vi "SQLite Backup Old Calibration Value.vi"(6 "backup/Delete":enum16{"Backup", "Delete"}(ring), 7 "Main":string="0", 8 "error in (no error)":errorcluster, 11 "VariableName":string) -> (0 "error out":errorcluster)   [LabVIEW 2017, in "SQLite.lvclass"]
doc: "保存校准的结果值,.\n2015-11-03 16:29:50\nBy：蒋松\nEmail：jiangsong@outlook.com\nSina: @sushu1051"
uses:
  SQLite.lvclass
  SQLiteFileName.ctl
  TabelFullName.ctl
  <vilib>/Utility/error.llb/Trim Whitespace.vi
  <userlib>/_OpenG.lib/array/array.llb/Remove Duplicates from 1D Array (String)__ogtk.vi
  <userlib>/LabSQL/LabSQL.lvlib
panel:
  out "Result Set":string[][](table) caption="Result Set (from first statement with results)"
  # "insert 之前要先删除所有的就的校准值。\n2015-11-03 16:45:40\nBy：蒋松\nEmail：jiangsong@outlook.com\nSina: @sushu1051"
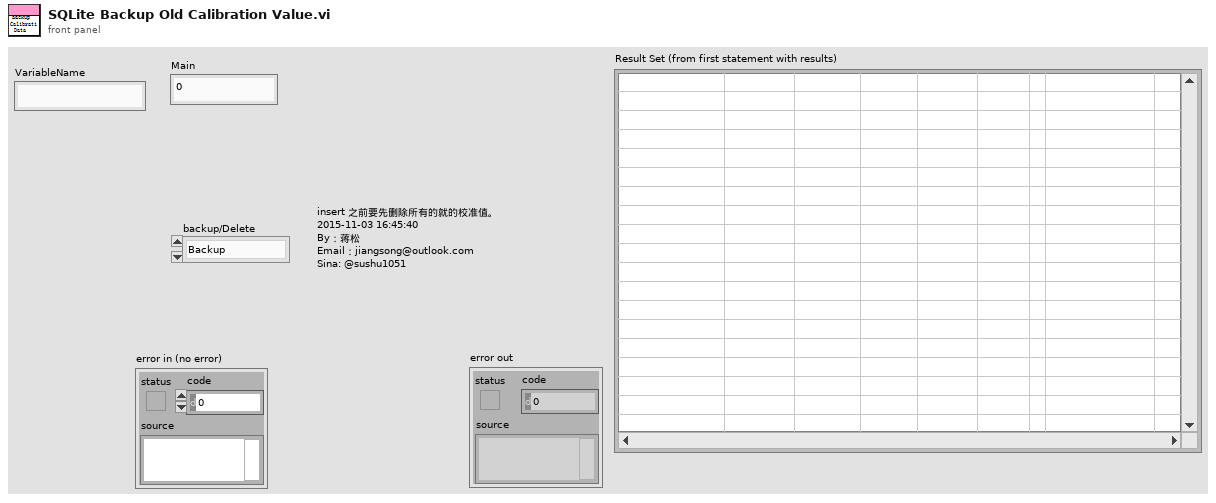
[diagram p1: front panel]
types:
  T1 = typedef "SQLite.lvclass/TabelFullName.ctl" = string
  T2 = typedef "SQLite.lvclass/SQLiteFileName.ctl" = string
  T3 = enum32{"invalid app kind", "Development System", "Run Time System", "Student Edition", "Embedded LabVIEW", "Evaluation", "Custom"}
  T4 = enum32{"Invalid", "Standard", "Closed", "Hidden", "Minimized", "Maximized"}
  T5 = enum16{"Other", "SQL2008", "SQLite", "Access", "MySQL"}
  T6 = cluster{"Core":cluster{"Current VI Reference":refnum<vi>, "Close Panel on Exit?":bool}}
  T7 = cluster{"Current VI Reference":refnum<vi>, "Close Panel on Exit?":bool}
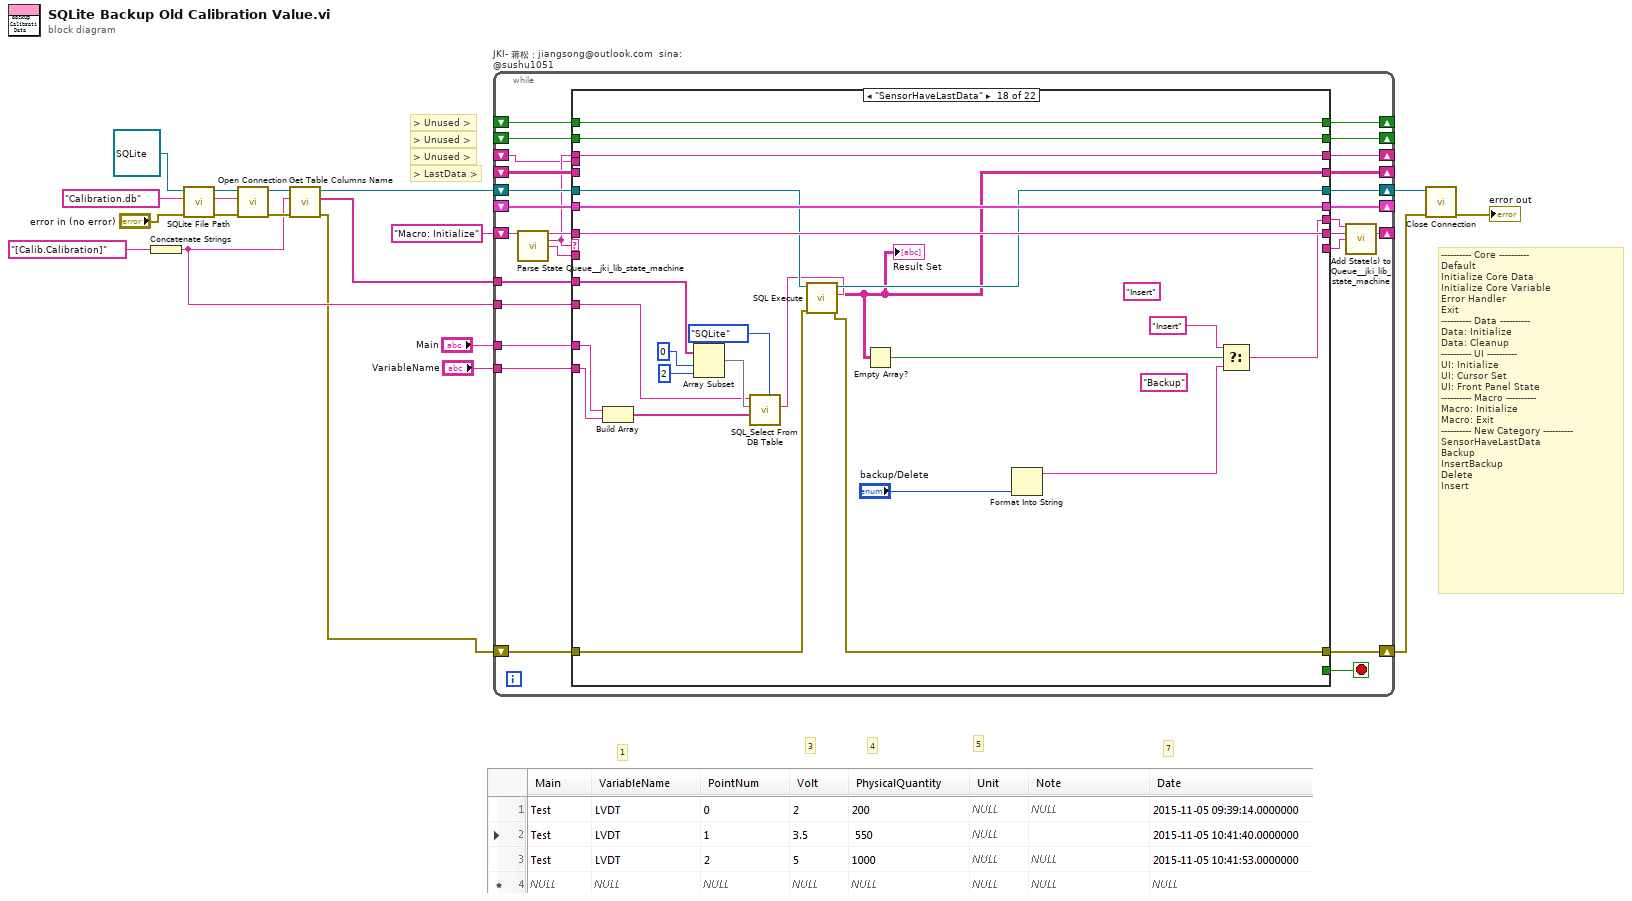
[diagram p0: block diagram]
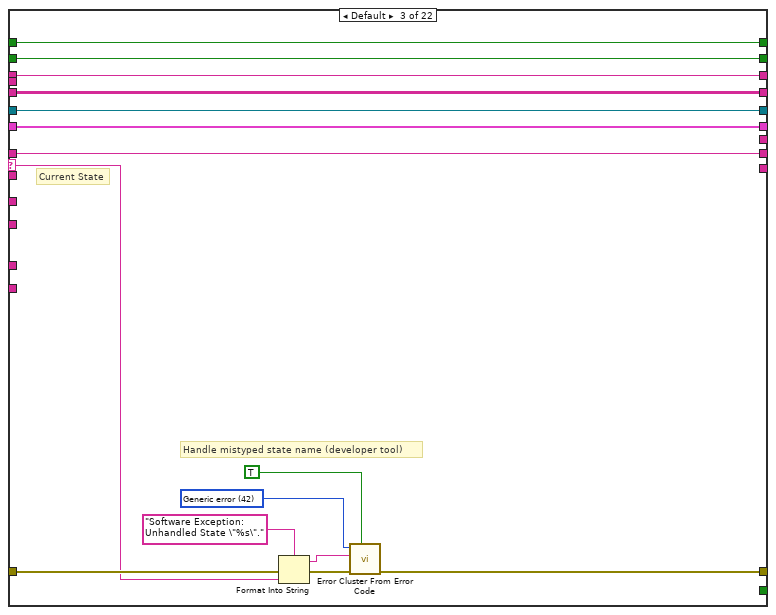
[diagram p4: hidden frame]
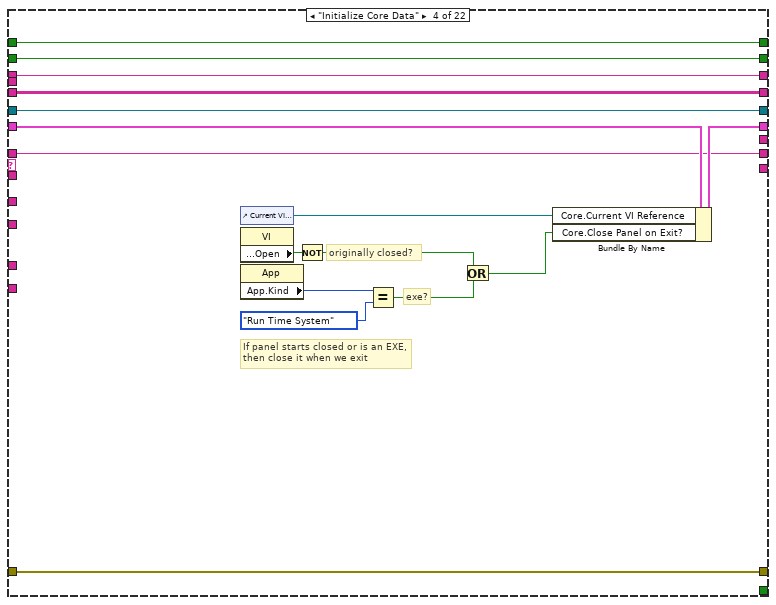
[diagram p5: hidden frame]
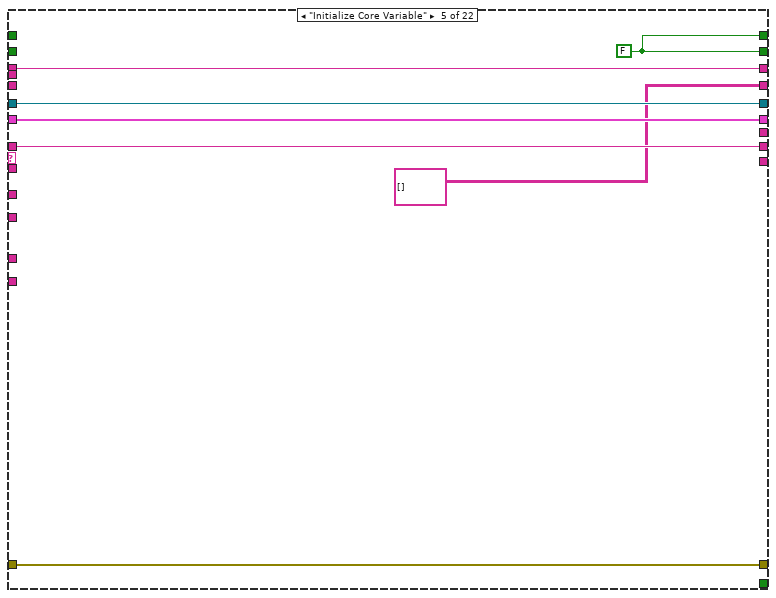
[diagram p6: hidden frame]
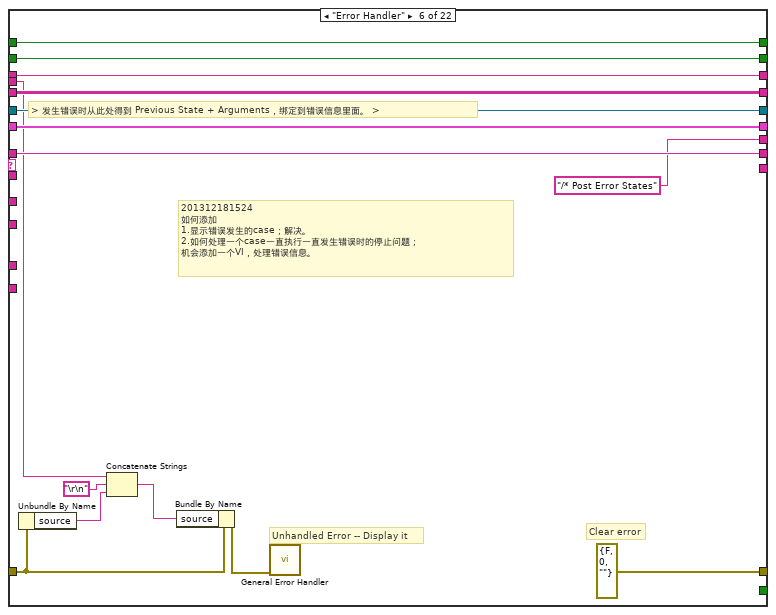
[diagram p7: hidden frame]
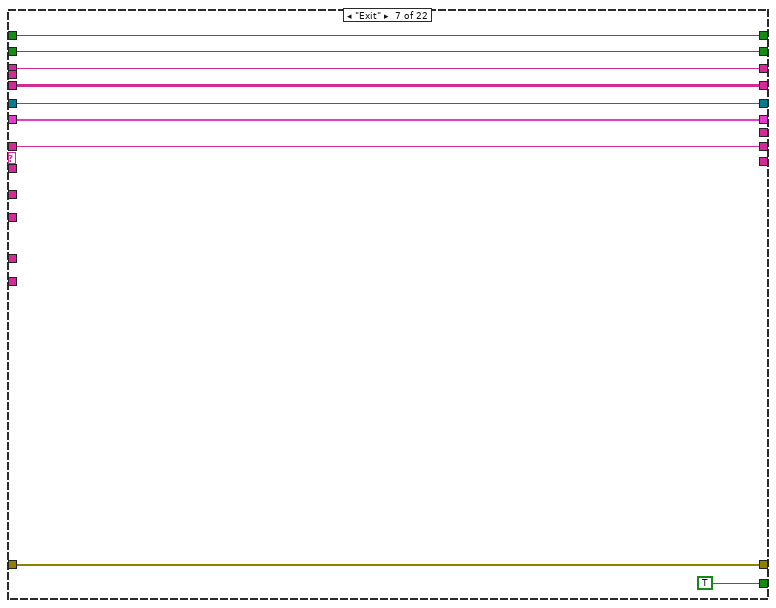
[diagram p8: hidden frame]
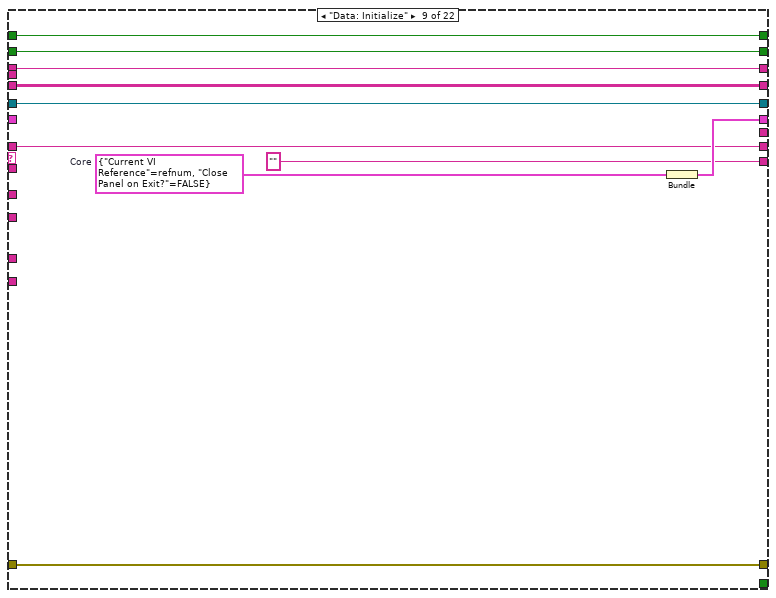
[diagram p10: hidden frame]
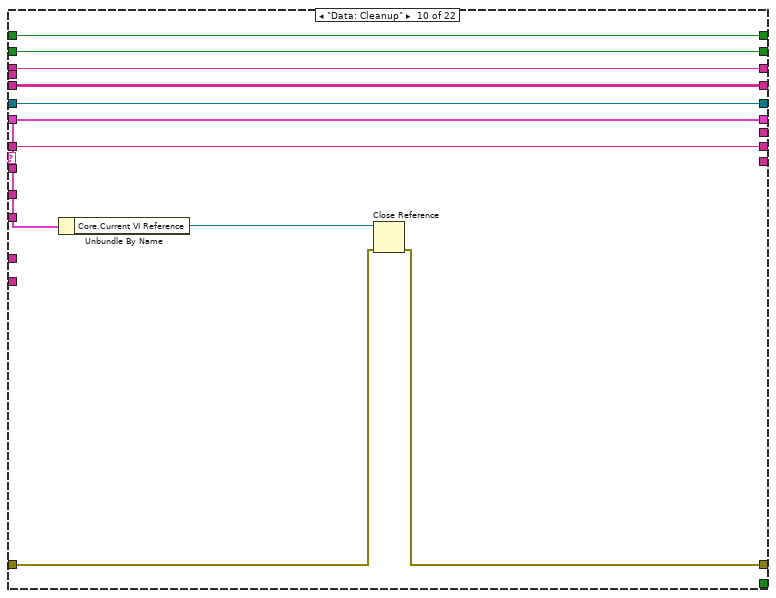
[diagram p11: hidden frame]
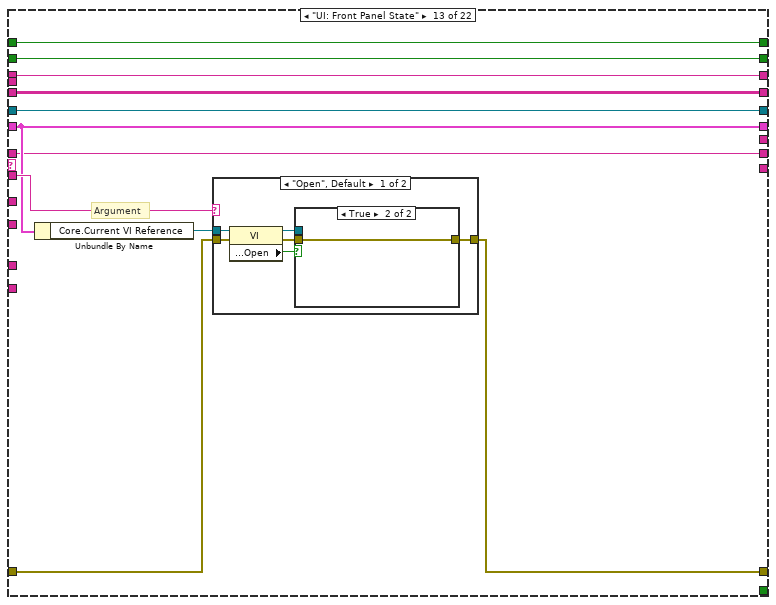
[diagram p14: hidden frame]
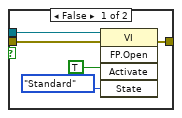
[diagram p15: hidden frame]
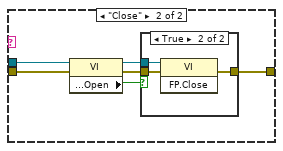
[diagram p16: hidden frame]
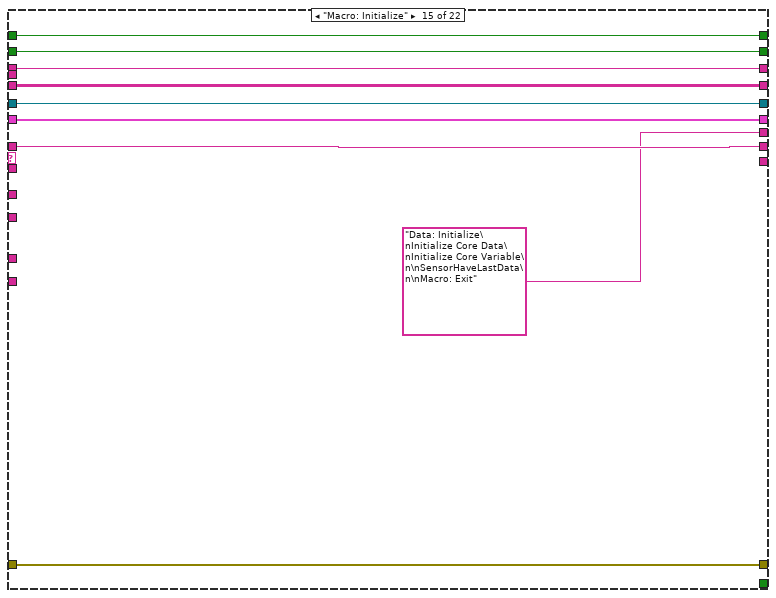
[diagram p19: hidden frame]
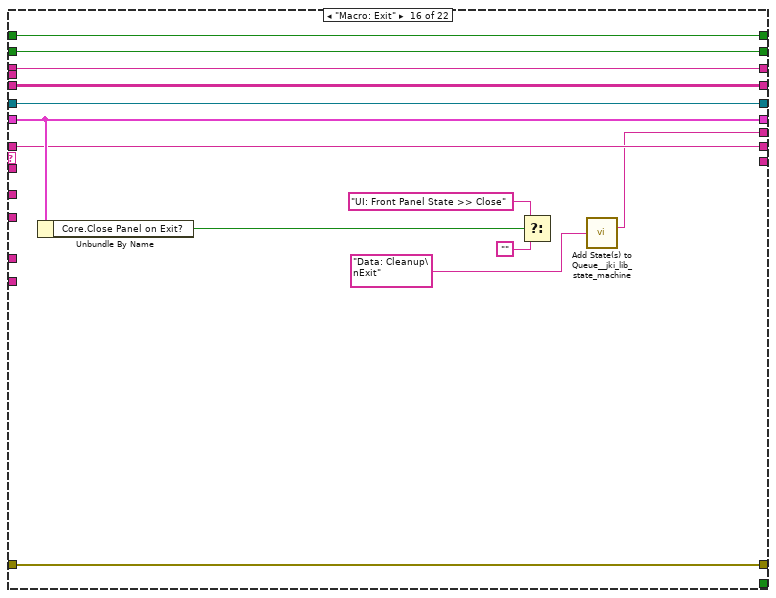
[diagram p20: hidden frame]
diagram:
  # "1"
  # "7"
  # "5"
  # "4"
  # "3"
  # "> Unused >"
  # "> LastData >"
  # "> Unused >"
  # "> Unused >"
  # "---------- Core ----------\nDefault\nInitialize Core Data\nInitialize Core Variable\nError Handler\nExit\n---------- Data ----------\nData: Initialize\nData: Cleanup\n---------- UI ----------\nUI: Initialize\nUI: Cursor Set\nUI: Front Panel State\n---------- Macro ----------\nMacro: Initialize\nMacro: Exit\n---------- New Category ----------\nSensorHaveLastData\nBackup\nInsertBackup\nDelete\nInsert"
  n1 = Concatenate Strings(T1 "[Calib.Calibration]" ("TabelFullName")) -> (w6:string)
  n2 = call "SQLite File Path.vi"("error in (no error)"="error in (no error)", "SQLiteFileName"=T2 "Calibration.db", "SQLite in"=refnum<class "SQLite.lvclass"> refnum ("SQLite.lvclass")) -> ("error out"=w16:errorcluster, "string"=w11:string, "SQLite out"=w13:refnum<class "SQLite.lvclass">)  [unwired: 6 in]
  n3 = call-dynamic "Open Connection.vi"("error in (no error)"=w16, "ConnectionString"=w11, "HostDB in"=w13) -> ("error out"=w10:errorcluster, "HostDB out"=w9:refnum<class "SQLite.lvclass">)  [unwired: 7 in]
  n4 = call-dynamic "Get Table Columns Name.vi"("error in (no error)"=w10, "TableName"=w6, "HostDB in"=w9) -> ("error out"=w5:errorcluster, "ColunmsList"=w7:string[], "HostDB out"=w8:refnum<class "SQLite.lvclass">)  [unwired: 4 in, 2 out]
  n5 = while "JKI- 蒋松：jiangsong@outlook.com  sina: @sushu1051" {
    shift-right: [w44] -> w2
    shift-left: w5 -> [w42]
    shift-right: [w32] -> _
    shift-left: "Macro: Initialize" -> [w33]
    shift-right: [w39] -> _
    shift-left: _ -> [w20]
    shift-right: [w40] -> _
    shift-left: _ -> [w41]
    shift-right: [w34] -> _
    shift-left: _ -> [w37]
    shift-right: [w35] -> w3
    shift-left: w8 -> [w28]
    shift-right: [w36] -> _
    shift-left: _ -> [w38]
    shift-right: [w27] -> _
    shift-left: _ -> [w26]
    tunnel: w7 -> [w25]
    tunnel: w6 -> [w24]
    tunnel: "Main" -> [w23]
    tunnel: "VariableName" -> [w22]
    stop <- w43 stop-if-true
    n6 = call <vilib>:"Parse State Queue__jki_lib_state_machine.vi"("State Queue"=w33) -> ("Remaining States"=w46:string, "Current State"=w21:string, "Arguments"=w45:string)  [unwired: 11 in, 1 out]
    n7 = case shown="\"SensorHaveLastData\"" w21 {
      selector: w21 -> [_ _ w65 _ _ _ _ _ _ _ _ _ _ _ _ _ _ _ _ _ _ _]
      tunnel: w46 -> [w54 w56 w64 w79 w98 w105 w117 w126 w135 w144 w154 w162 w170 w203 w212 w221 w233 w261 w299 w321 w340 w347]
      tunnel: w45 -> [_ _ _ _ _ _ _ _ _ _ _ _ w173 _ _ _ _ _ _ _ _ _]
      tunnel: [w53 w62 w66 w90 w100 errorcluster {"status"=FALSE, "code"=0, "source"=""} ("error out") w119 w128 w139 w146 w156 w164 w174 w205 w214 w228 w236 w243 w267 w304 w333 w348] -> w44
      tunnel: w42 -> [w53 w62 w67 w90 w100 w109 w119 w128 w139 w147 w156 w164 w175 w205 w214 w228 w236 w244 w268 w313 w331 w348]
      tunnel: [w54 w56 w64 w79 w98 w105 w117 w126 w135 w144 w154 w162 w170 w203 w212 w221 w233 w261 w299 w321 w340 w347] -> w31
      tunnel: [_ _ _ _ _ _ TRUE _ _ _ _ _ _ _ _ _ _ _ _ _ _ _] -> w43
      tunnel: w41 -> [w52 w61 w77 w93 _ w115 w124 w132 w142 w152 w160 w168 w179 w209 w218 w231 w239 w264 w302 w320 w339 w346]
      tunnel: w21 -> [w51 w60 w76 w92 w94 w114 w123 w131 w141 w151 w159 w167 w178 w208 w217 w230 w238 w263 w301 w319 w338 w345]
      tunnel: [w52 w61 w77 w93 w97 w115 w124 w132 w142 w152 w160 w168 w179 w209 w218 w231 w239 w264 w302 w320 w339 w346] -> w40
      tunnel: [w51 w60 w76 w92 w94 w114 w123 w131 w141 w151 w159 w167 w178 w208 w217 w230 w238 w263 w301 w319 w338 w345] -> w39
      tunnel: w38 -> [w50 w59 w75 w91 _ w113 w122 w130 w140 w150 w158 w166 w177 w207 w216 w229 w237 _ w280 w308 w335 w344]
      tunnel: w28 -> [w48 w57 w74 w80 w96 w103 w118 w127 w136 w145 w155 w163 w171 w204 w213 w222 w234 w248 w272 w316 w332 w343]
      tunnel: w37 -> [w49 w58 w73 w82 w99 w112 w121 w129 _ w148 w157 w165 w172 w206 w215 w223 w235 w262 w300 w318 w337 w342]
      tunnel: [w50 w59 w75 w91 string[][] [] ("Result Set") w113 w122 w130 w140 w150 w158 w166 w177 w207 w216 w229 w237 w245 w274 w308 w335 w344] -> w36
      tunnel: [w48 w57 w74 w80 w96 w103 w118 w127 w136 w145 w155 w163 w171 w204 w213 w222 w234 w247 w271 w315 w332 w343] -> w35
      tunnel: [w49 w58 w73 w81 w99 w112 w121 w129 w137 w148 w157 w165 w172 w206 w215 w223 w235 w262 w300 w318 w337 w342] -> w34
      tunnel: [_ _ _ _ _ "/* Post Error States" _ _ _ _ _ _ _ _ "Data: Initialize\nInitialize Core Data\nInitialize Core Variable\n\nSensorHaveLastData\n\nMacro: Exit" w220 _ w249 "InsertBackup" ("Remaining States") _ _ _] -> w30
      tunnel: [_ _ _ _ _ _ _ _ "" _ _ _ _ _ _ _ _ _ _ _ _ _] -> w29
      tunnel: w26 -> [w47 w55 w63 w78 _ w102 w116 w125 w133 w143 w153 w161 w169 w202 w210 w219 w232 w260 w298 w317 w336 w341]
      tunnel: [w47 w55 w63 w78 w97 w102 w116 w125 w133 w143 w153 w161 w169 w202 w210 w219 w232 w260 w298 w317 w336 w341] -> w27
      tunnel: w25 -> [_ _ _ _ _ _ _ _ _ _ _ _ _ _ _ _ _ w256 w291 w312 _ _]
      tunnel: w24 -> [_ _ _ _ _ _ _ _ _ _ _ _ _ _ _ _ _ w255 w294 w314 _ _]
      tunnel: w23 -> [_ _ _ _ _ _ _ _ _ _ _ _ _ _ _ _ _ w252 _ _ _ _]
      tunnel: w22 -> [_ _ _ _ _ _ _ _ _ _ _ _ _ _ _ _ _ w253 w292 w306 w334 _]
      tunnel: w20 -> [_ _ _ _ _ w101 _ _ _ _ _ _ _ _ _ _ _ _ _ _ _ _]
      frame "Idle" {
      }
      frame "---------- Core ----------" {
      }
      frame Default {
        w69 = 42 items=["No error", "Argument error", "Memory is full", "Out of zone", "End of file", "File already open", "Generic file I/O error", "File not found", "File permission error", "Disk is full", "Duplicate path", "Too many files open", "System feature not enabled", "Resource file not found", "Cannot add resource", "Resource not found", "Image not found", "Image memory error", "Pen does not exist", "Config type invalid", "Config token not found", "Config parse error", "Config memory error", "Bad external code format", "Bad external code offset", "External code not present", "Null window", "Destroy window error", "Null menu", "Print aborted", "Bad print record", "Print driver error", "Windows error during printing", "Memory error during printing", "Print dialog error", "Generic print error", "Invalid device refnum", "Device not found", "Device parameter error", "Device unit error", "Cannot open device", "Device call aborted", "Generic error", "Cancelled by user", "Object ID too low", "Object ID too high", "Object not in heap", "Unknown heap", "Unknown object (invalid DefProc)", "Unknown object (DefProc not in table)", "Message out of range", "Invalid (null) method", "Unknown message", "Manager call not supported", "Bad address", "Network operation in progress", "Network operation timed out", "Connection is busy", "Network attribute not supported", "Network error", "Address in use", "System out of memory", "Connection aborted", "Connection refused", "Not connected", "Already connected", "Connection closed", "Initialization error (interapplication manager)", "Bad occurrence", "Wait on unbound occurrence handler", "Occurrence queue overflow", "Datalog type conflict", "Unused", "Unrecognized type (interapplication manager)", "Memory corrupt", "Failed to make temporary DLL", "Old CIN version", "Drag socket not found", "Failed to load drop-object", "Failed to register OLE object", "Failed to release OLE object", "Format specifier type mismatch", "Unknown format specifier", "Too few format specifiers", "Too many format specifiers", "Scan failed", "Newer CIN version", "Error converting to variant", "Runtime menu error", "Password tampered", "Variant attribute not found", "Incompatible variant data type", "Event data is not available", "Event Store is not present", "Occurrence is not found", "Event Queue is not created", "Event info is not available", "Refnum passed is NULL", "Error retrieving Class GUID", "Error retrieving CoClass GUID", "Error retrieving TypeLib GUID.", "Bad built application magic bytes.", "Specific driver is different from the specific driver associated with the Logical Name.", "There is no session opened to the class driver.", "Max Error", "MAX - Error with config objects", "MAX - Error loading configuration", "MAX - Group not supported"]
        # "Current State"
        # "Handle mistyped state name (developer tool)"
        n8 = Format Into String(format string="Software Exception: Unhandled State \"%s\"." ("message"), error in=w67, w65) -> (resulting string=w70:string, error out=w71:errorcluster)  [unwired: 1 in]
        n9 = call <vilib>:"Error Cluster From Error Code.vi"("show call chain? (False)"=TRUE, "error in (no error)"=w71, "error message (\"\")"=w70, "error code (0)"=w69) -> ("error out"=w66:errorcluster)  [unwired: 5 in]
      }
      frame "Initialize Core Data" {
        # "originally closed?"
        # "exe?"
        # "If panel starts closed or is an EXE, then close it when we exit"
        n10 = control-ref of="Current VI Reference"() -> (w89:refnum<vi>)
        n11 = property class="VI"() -> ("Front Panel.Open"=w83:bool)  [unwired: 2 in, 2 out]
        n12 = property class="App"() -> ("App.Kind"=w84:T3)  [unwired: 2 in, 2 out]
        n13 = Not(x=w83) -> (.not. x?=w86:bool)
        n14 = Equal?(x=w84, y=T3."Run Time System" ("Application:Kind")) -> (x = y?=w87:bool)
        n15 = Or(x=w86, y=w87) -> (x .or. y?=w88:bool)
        n16 = Bundle By Name(cluster=w82, "Core.Current VI Reference"=w89, "Core.Close Panel on Exit?"=w88) -> (w81:T6)
      }
      frame "Initialize Core Variable" {
        w97 = FALSE
      }
      frame "Error Handler" {
        # "> 发生错误时从此处得到 Previous State + Arguments，绑定到错误信息里面。 >"
        # "201312181524\n如何添加\n1.显示错误发生的case；解决。\n2.如何处理一个case一直执行一直发生错误时的停止问题；\n机会添加一个VI，处理错误信息。"
        # "Clear error"
        # "Unhandled Error -- Display it"
        n17 = Unbundle By Name(w109) -> ("source"=w107:string)
        n18 = Concatenate Strings(w101, "\r\n", w107) -> (w106:string)
        n19 = Bundle By Name(cluster=w109, "source"=w106) -> (w110:errorcluster)
        n20 = call <vilib>:"General Error Handler.vi"("error in (no error)"=w110) -> ()  [unwired: 10 in, 5 out]
      }
      frame "Exit" {
      }
      frame "---------- Data ----------" {
      }
      frame "Data: Initialize" {
        w138 = T7 {"Current VI Reference"=refnum, "Close Panel on Exit?"=FALSE}  # Core
        n21 = Bundle("Core"=w138) -> (w137:T6)  [unwired: 1 in]
      }
      frame "Data: Cleanup" {
        n22 = Unbundle By Name(w148) -> ("Core.Current VI Reference"=w149:refnum<vi>)
        n23 = Close Reference(reference=w149, error in (no error)=w147) -> (error out=w146:errorcluster)
      }
      frame "---------- UI ----------" {
      }
      frame "UI: Initialize" {
      }
      frame "UI: Front Panel State" {
        # "Argument"
        n24 = Unbundle By Name(w172) -> ("Core.Current VI Reference"=w176:refnum<vi>)
        n25 = case shown="\"Open\", Default" w173 {
          tunnel: w175 -> [w183 w196]
          tunnel: [w185 w197] -> w174
          tunnel: w176 -> [w184 w194]
          frame "Open", Default {
            n26 = property class="VI"(reference=w184, error in=w183) -> (reference out=w181:refnum<vi>, error out=w182:errorcluster, "Front Panel.Open"=w180:bool)
            n27 = case shown="True" w180 {
              tunnel: [w188 w191] -> w185
              tunnel: w182 -> [w187 w191]
              tunnel: w181 -> [w186 _]
              frame False {
                n28 = invoke class="VI" method="FP.Open"(reference=w186, error in=w187, "Activate"=TRUE, "State"=T4."Standard") -> (error out=w188:errorcluster)  [unwired: 1 in, 4 out]
              }
              frame True {
              }
            }
          }
          frame "Close" {
            n29 = property class="VI"(reference=w194, error in=w196) -> (reference out=w193:refnum<vi>, error out=w195:errorcluster, "Front Panel.Open"=w192:bool)
            n30 = case shown="True" w192 {
              tunnel: [w198 w201] -> w197
              tunnel: w195 -> [w198 w200]
              tunnel: w193 -> [_ w199]
              frame False {
              }
              frame True {
                n31 = invoke class="VI" method="FP.Close"(reference=w199, error in=w200) -> (error out=w201:errorcluster)  [unwired: 1 in, 2 out]
              }
            }
          }
        }
      }
      frame "---------- Macro ----------" {
      }
      frame "Macro: Initialize" {
      }
      frame "Macro: Exit" {
        n32 = Unbundle By Name(w223) -> ("Core.Close Panel on Exit?"=w224:bool)
        n33 = Select(t="UI: Front Panel State >> Close", s=w224, f="") -> ()  [unwired: 1 out]
        n34 = call <vilib>:"Add State(s) to Queue__jki_lib_state_machine.vi"("State(s) at Back (\"\")"="Data: Cleanup\nExit") -> ("States Out"=w220:string)  [unwired: 14 in]
      }
      frame "---------- New Category ----------" {
      }
      frame "SensorHaveLastData" {
        (unwired) "Insert" ("Remaining States")
        (unwired) "Backup" ("Remaining States")
        n35 = Build Array(w252, w253) -> (w254:string[])
        n36 = Array Subset(array=w256, index=0, length=2) -> (w258:string[])
        n37 = call <userlib>:"SQL_Select From DB Table.vi"("DB Type"=T5."SQLite", "ColumnsValue"=w254, "ColumnsNameList"=w258, "TableName"=w255) -> ("Select SQL CMD"=w246:string)  [unwired: 7 in]
        n38 = call-dynamic "SQL Execute.vi"("error in (no error)"=w244, "Command Text"=w246, "HostDB in"=w248) -> ("error out"=w243:errorcluster, "Table Control"=w245:string[][], "HostDB out"=w247:refnum<class "SQLite.lvclass">)  [unwired: 4 in, 2 out]
        "Result Set" <- w245
        n39 = Empty Array?(array=w245) -> (empty?=w251:bool)
        n40 = Format Into String("backup/Delete") -> (resulting string=w241:string)  [unwired: 3 in, 1 out]
        n41 = Select(t="Insert" ("Remaining States"), s=w251, f=w241) -> (s? t:f=w249:string)
      }
      frame "Backup" {
        # "get Main Max ,and add1 for backup data.\n2016-08-29 14:38:51"
        n42 = Build Array(w292) -> (w293:string[])
        n43 = Array Subset(array=w291, index=1, length=1) -> (w296:string[])
        n44 = Index Array(array=w291, index=0) -> (element=w289:string)
        n45 = Build Array(w289) -> (w288:string[])
        n46 = call <userlib>:"SQL_Select From DB Table.vi"("DB Type"=T5."SQLite", "SelectedColumnsNameList"=w288, "ColumnsValue"=w293, "ColumnsNameList"=w296, "TableName"=w294) -> ("Select SQL CMD"=w270:string)  [unwired: 6 in]
        n47 = call-dynamic "SQL Execute.vi"("error in (no error)"=w268, "Return Data (T)"=TRUE, "Command Text"=w270, "HostDB in"=w272) -> ("error out"=w267:errorcluster, "Table Control"=w269:string[][], "HostDB out"=w271:refnum<class "SQLite.lvclass">)  [unwired: 3 in, 2 out]
        n48 = Index Array(array=w269, index (col)=0 ("disabled index (col)")) -> (element=w287:string[])  [unwired: 1 in]
        n49 = call-poly <userlib>:"Remove Duplicates from 1D Array__ogtk.vi"("Input Array"=w287) -> ("Output Array"=w285:string[])  [unwired: 1 out]
        n50 = Decimal String To Number(string=w285) -> (number=w284:i32[])  [unwired: 2 in, 1 out]
        n51 = Array Max & Min(array=w284) -> (max value=w283:i32)  [unwired: 3 out]
        n52 = Array Size(array=w280) -> (size(s)=w279:i32[])
        n53 = Increment(x=w283) -> (x+1=w282:i32)
        n54 = Number To Decimal String(number=w282) -> (decimal integer string=w276:string)  [unwired: 1 in]
        n55 = Index Array(array=w279, index=0) -> (element=w277:i32)
        n56 = Initialize Array(w276, w277) -> (w275:string[])
        n57 = Replace Array Subset(array=w280, new element=w275, index (col)=0 ("disabled index (col)")) -> (w274:string[][])  [unwired: 1 in]
      }
      frame "InsertBackup" {
        w309 = 6 ("length")
        w310 = 0 ("index")
        n58 = Array Subset(array=w312, index=w310, length=w309) -> (w311:string[])
        n59 = Array Subset(array=w308, index (col)=w310, length (col)=w309) -> (w307:string[][])  [unwired: 2 in]
        n60 = for {
          tunnel: w314 -> [w330]
          tunnel: w311 -> [w329]
          shift-right: [w326] -> w315
          shift-left: w316 -> [w327]
          shift-right: [w323] -> w305
          shift-left: w313 -> [w324]
          tunnel: w307 -> [w328] mode=indexing
          tunnel: enum16{"Other", "SQL2008", "SQLite"}."SQLite" ("DB Type") -> [w322]
          n61 = call <userlib>:"SQL_Insert DB Table.vi"("DB Type"=w322, "ColumnsValue"=w328, "ColumnsName"=w329, "Table Name"=w330) -> ("Insert DB String"=w325:string)  [unwired: 7 in]
          n62 = call-dynamic "SQL Execute.vi"("error in (no error)"=w324, "Command Text"=w325, "HostDB in"=w327) -> ("error out"=w323:errorcluster, "HostDB out"=w326:refnum<class "SQLite.lvclass">)  [unwired: 4 in, 3 out]
        }
        n63 = call "SQLite Delete All Calibration Data.vi"("error in (no error)"=w305, "VariableName"=w306) -> ("error out"=w304:errorcluster)  [unwired: 7 in, 2 out]
      }
      frame "Delete" {
        (unwired) enum16{"Other", "SQL2008", "SQLite"}."SQLite" ("DB Type")
        n64 = call "SQLite Delete All Calibration Data.vi"("error in (no error)"=w331, "VariableName"=w334) -> ("error out"=w333:errorcluster)  [unwired: 7 in, 2 out]
      }
      frame "Insert" {
      }
    }
    n65 = call <vilib>:"Add State(s) to Queue__jki_lib_state_machine.vi"("State(s) in Front (\"\")"=w30, "State(s) in (\"\")"=w31, "State(s) at Back (\"\")"=w29) -> ("States Out"=w32:string)  [unwired: 12 in]
  }
  n66 = call-dynamic "Close Connection.vi"("error in (no error)"=w2, "HostDB in"=w3) -> ("error out"=→"error out":errorcluster)  [unwired: 8 in, 1 out]
